vi "223 Crop Image.vi"(11 "Camera Image 2":T1) -> (3 "Cropped Image 2":T1)   [LabVIEW 2012]
uses:
  <vilib>/vision/Image Controls.llb/IMAQ Image.ctl
  <vilib>/vision/NI_Vision_Development_Module.lvlib
panel:
  in  "Left Percent":dbl=0.45
  in  "Right Percent":dbl=0.45
  in  "Top Percent":dbl=0.45
  in  "Bottom Percent":dbl=0.45
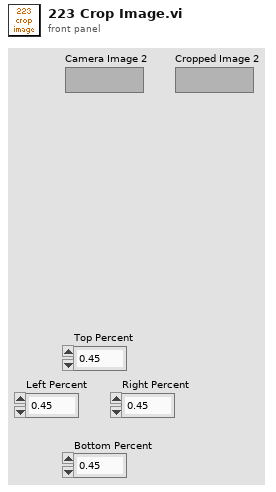
[diagram p1: front panel]
types:
  T1 = typedef "IMAQ Image.ctl" = refnum<image>
  T2 = typedef "Image Type" = u32
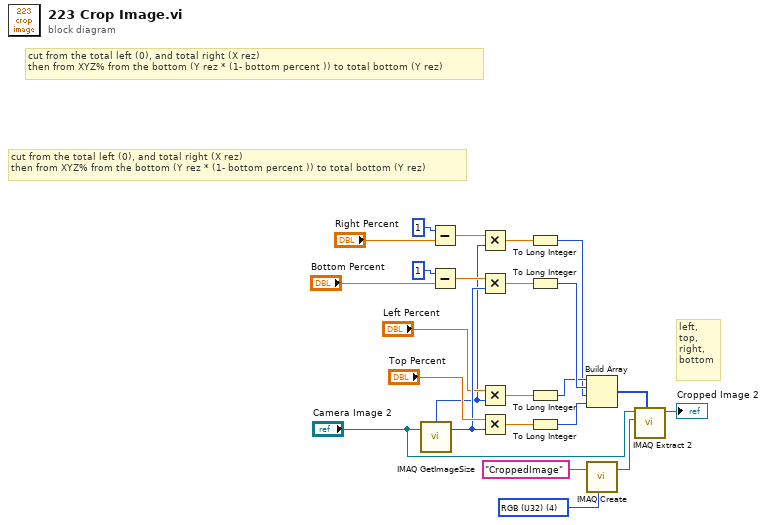
[diagram p0: block diagram]
diagram:
  w14 = T2 4 items=["Grayscale (U8)", "Grayscale (I16)", "Grayscale (SGL)", "Complex (CSG)", "RGB (U32)", "HSL (U32)", "RGB (U64)", "Grayscale (U16)"] ("Image Type")
  # "cut from the total left (0), and total right (X rez)\nthen from XYZ% from the bottom (Y rez * (1- bottom percent )) to total bottom (Y rez)"
  # "left, \ntop, \nright, \nbottom"
  # "cut from the total left (0), and total right (X rez)\nthen from XYZ% from the bottom (Y rez * (1- bottom percent )) to total bottom (Y rez)"
  n1 = call "IMAQ GetImageSize"("Image"="Camera Image 2") -> ("Y Resolution"=w10:i32, "X Resolution"=w3:i32)  [unwired: 3 in, 1 out]
  n2 = Subtract(x=1, y="Right Percent") -> (x-y=w7:dbl)
  n3 = Subtract(x=1, y="Bottom Percent") -> (x-y=w21:dbl)
  n4 = Multiply(x=w7, y=w3) -> (x*y=w6:dbl)
  n5 = Multiply(x=w21, y=w10) -> (x*y=w18:dbl)
  n6 = Multiply(x="Left Percent", y=w3) -> (x*y=w5:dbl)
  n7 = Multiply(x="Top Percent", y=w10) -> (x*y=w13:dbl)
  n8 = To Long Integer(number=w6) -> (32bit integer=w1:i32)
  n9 = To Long Integer(number=w18) -> (32bit integer=w20:i32)
  n10 = To Long Integer(number=w5) -> (32bit integer=w2:i32)
  n11 = To Long Integer(number=w13) -> (32bit integer=w11:i32)
  n12 = Build Array(w2, w20, w1, w11) -> (w19:i32[])
  n13 = call "IMAQ Create"("Image Name"="CroppedImage", "Image Type"=w14) -> ("New Image"=w16:T1)  [unwired: 3 in, 1 out]
  n14 = call "IMAQ Extract 2"("Optional Rectangle"=w19, "Image Dst"=w16, "Image Src"="Camera Image 2") -> ("Image Dst Out"=→"Cropped Image 2":T1)  [unwired: 7 in, 1 out]
